vi "Handle Error.vi"(8 "error in (no error)":errorcluster, 11 "InterferometryUI in":refnum<class "InterferometryUI.lvclass">) -> (0 "error out":errorcluster, 2 "stop actor?":bool=TRUE, 3 "InterferometryUI out":refnum<class "InterferometryUI.lvclass">)   [LabVIEW 2023, in "InterferometryUI.lvlib" / "InterferometryUI.lvclass"]
doc: "<p>(<strong>Filename</strong>: <span class=\"dnl\">Actor Framework.lvlib:Actor.lvclass:Handle Error.vi</span>)</p>\n<p>Defines how the actor handles an error that occurred while processing a message. By default, this method does nothing except stop the actor.</p>"
uses:
  InterferometryUI.lvclass
  <vilib>/ActorFramework/Actor/Actor.lvclass
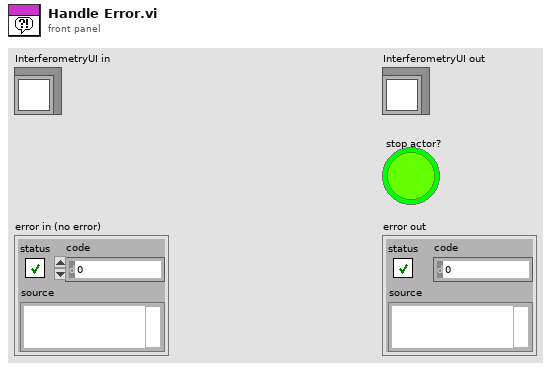
[diagram p1: front panel]
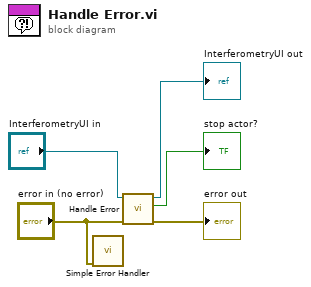
[diagram p0: block diagram]
diagram:
  n1 = call <vilib>:"Simple Error Handler.vi"("error in (no error)"="error in (no error)") -> ()  [unwired: 4 in, 5 out]
  n2 = call-parent "Handle Error.vi"("error in (no error)"="error in (no error)", "Actor in"="InterferometryUI in") -> ("error out"=→"error out":errorcluster, "stop actor?"=→"stop actor?":bool, "Actor out"=→"InterferometryUI out":refnum<class "InterferometryUI.lvclass">)  [unwired: 7 in]
